vi "Write Field (Variant).vi"(7 "field name":string, 8 "error in (no error)":errorcluster, 10 "value in":variant, 11 "PV Data in":refnum<class "PV Data.lvclass">) -> (0 "error out":errorcluster, 2 "value out":variant, 3 "PV Data out":refnum<class "PV Data.lvclass">)   [LabVIEW 2020, in "PV Access.lvlib" / "PV Data.lvlib" / "PV Data.lvclass"]
uses:
  PV Data.lvclass
  <vilib>/ErrorRing/Error Ring.xnode
  PV Data.lvclass/PV Data.ctl
  cceb9e4b-eb75-48e8-aa55-ce9bdc72e988.vi
  c2285a35-9ffd-4e7b-9c27-aea24fb1581d.vi
  9a7adfbc-dfd7-46c4-b075-4f0440b83174.vi
  1bea9b6c-c326-4b2e-8e3d-45bf733a9c38.vi
  d9fbc47b-4e38-408d-93dd-f03e8c927dfc.vi
  878da8d4-af84-4ac8-b8bd-4e3d6f536ca0.vi
  22b99ade-ebf6-47b9-88b0-a2a84584e77c.vi
  7938dc55-06bb-4f46-98b4-31ec94e48f5a.vi
  17bcbbb4-445b-4ae2-9ca0-bb438421ceb4.vi
  76e53dd5-f0c3-4a89-968d-82371d9cf6ec.vi
  9c6bba7f-697c-4d5e-a550-b75ffba85a50.vi
  02c85caf-8b62-432b-a175-5fdc5c038fcc.vi
  5a5bdb7c-77ef-45fb-97e8-dbe02cadd076.vi
  b370053f-91cb-4be5-8525-cb241afcd6fe.vi
  a549df2c-920d-4323-ba7c-d4da420400e8.vi
  79192ce2-8dd6-4a70-8822-a4eb65a6aaee.vi
  1431eaa6-23a1-45b9-a4a3-2693041a1402.vi
  05adf883-15cd-45cb-9d7e-7746134da8fa.vi
  2414d7e0-05f5-4190-ab07-d4c7ba67c6a6.vi
  efa8a1d7-3bed-4705-901c-3918d28cffa5.vi
  26f11cd7-ec94-4004-9a33-110acaed2e3e.vi
  cc62e3b5-8986-4e79-a38c-535dac47f5c9.vi
  21c48d27-f92c-4ff3-9f7e-da22303d9520.vi
  0dfc8336-85bc-4349-aa6f-77eea7d3ae68.vi
  PV Data.lvlib
  <vilib>/Utility/Data Type/NI_Data Type.lvlib
  <vilib>/Utility/error.llb/Error Cluster From Error Code.vi
  Write Field (Boolean).vi
  Write Field (Boolean Array).vi
  Write Field (I8).vi
  Write Field (I8 Array).vi
  Write Field (I16).vi
  Write Field (I16 Array).vi
  Write Field (I32).vi
  Write Field (I32 Array).vi
  Write Field (I64).vi
  Write Field (I64 Array).vi
  Write Field (U8).vi
  Write Field (U8 Array).vi
  Write Field (U16).vi
  Write Field (U16 Array).vi
  Write Field (U32).vi
  Write Field (U32 Array).vi
  Write Field (U64).vi
  Write Field (U64 Array).vi
  Write Field (SGL).vi
  Write Field (DBL).vi
  Write Field (SGL Array).vi
  Write Field (DBL Array).vi
  Write Field (String).vi
  Write Field (String Array).vi
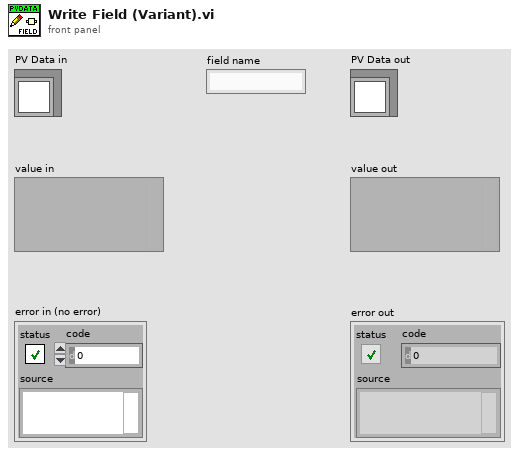
[diagram p1: front panel]
types:
  T1 = typedef "NI_Data Type.lvlib/Data Type.ctl" = enum8{"Invalid Type", "Void", "I8", "I16", "I32", "I64", "U8", "U16", "U32", "U64", "Single Float", "Double Float", "Extended Float", "Single Complex", "Double Complex", "Extended Complex", "Enum U8", "Enum U16", "Enum U32", "Enum U64", "Single Float With Unit", "Double Float With Unit", "Extended Float With Unit", "Single Complex with Unit", "Double Complex with Unit", "Extended Complex with Unit", "Boolean", "String", "Path", "Picture", "Tag", "Array", "Cluster", "Variant", "LV Variant", "Waveform", "Timestamp", "Digital Waveform", "Digital Data", "ExpressData", "Refnum", "External Data", "VI", "Poly VI", "LabVIEW Class Instance", "Fixed Point", "Set Collection", "Map Collection"}
  T2 = typedef "PV Access.lvlib/PV Data.lvlib/Type Code.ctl" = enum8{"Null", "Bool", "BoolA", "Int8", "Int8A", "Int16", "Int16A", "Int32", "Int32A", "Int64", "Int64A", "UInt8", "UInt8A", "UInt16", "UInt16A", "UInt32", "UInt32A", "UInt64", "UInt64A", "Float32", "Float32A", "Float64", "Float64A", "String", "StringA", "Struct", "StructA", "Union", "UnionA", "Any", "AnyA"}
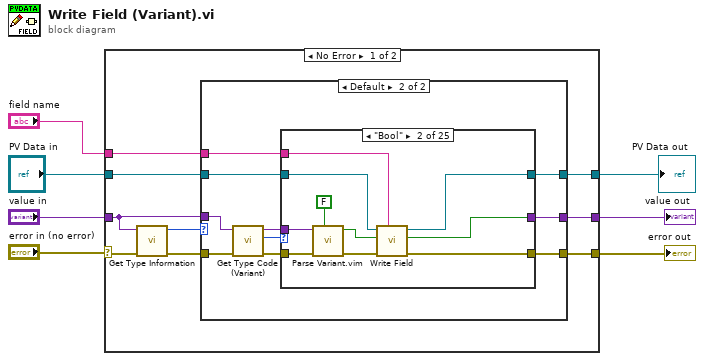
[diagram p0: block diagram]
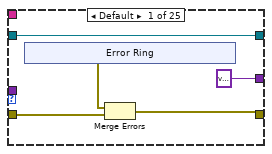
[diagram p3: hidden frame]
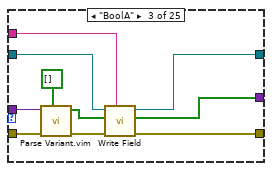
[diagram p4: hidden frame]
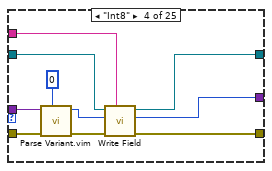
[diagram p5: hidden frame]
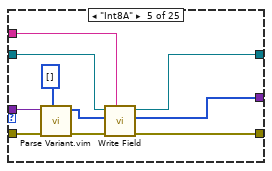
[diagram p6: hidden frame]
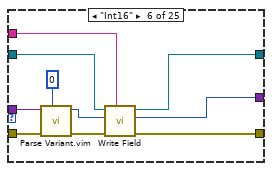
[diagram p7: hidden frame]
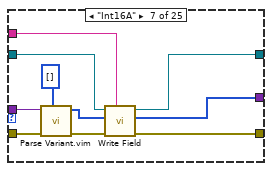
[diagram p8: hidden frame]
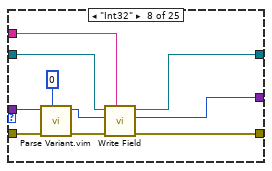
[diagram p9: hidden frame]
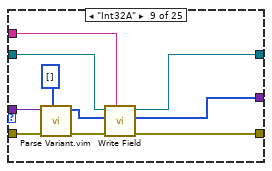
[diagram p10: hidden frame]
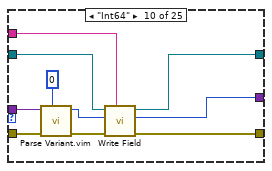
[diagram p11: hidden frame]
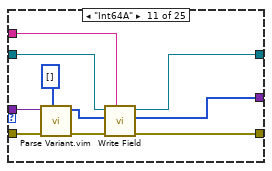
[diagram p12: hidden frame]
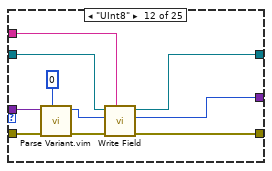
[diagram p13: hidden frame]
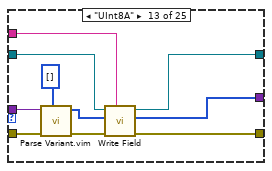
[diagram p14: hidden frame]
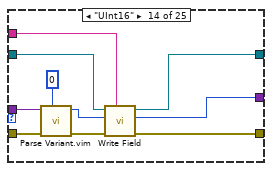
[diagram p15: hidden frame]
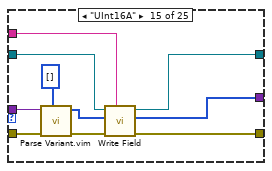
[diagram p16: hidden frame]
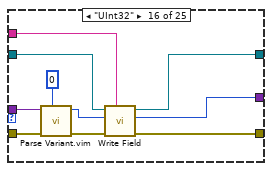
[diagram p17: hidden frame]
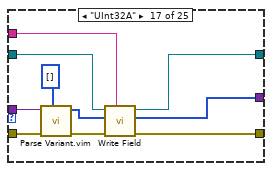
[diagram p18: hidden frame]
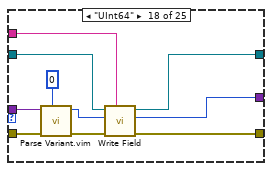
[diagram p19: hidden frame]
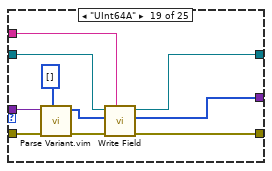
[diagram p20: hidden frame]
diagram:
  n1 = case shown="No Error" "error in (no error)" {
    selector: "error in (no error)" -> [w10 w279]
    tunnel: "value in" -> [w11 w280]
    tunnel: [w16 w280] -> w5
    tunnel: [w15 w279] -> w4
    tunnel: "PV Data in" -> [w14 w281]
    tunnel: [w13 w281] -> w2
    tunnel: "field name" -> [w12 _]
    frame No Error {
      n2 = call <vilib>:"Get Type Information.vi"("error in (no error)"=w10, "variant"=w11) -> ("error out"=w9:errorcluster, "type"=w8:T1)  [unwired: 5 in, 3 out]
      n3 = case shown="Default" w8 {
        tunnel: [w19 w26] -> w16
        tunnel: [w18 w25] -> w15
        tunnel: w14 -> [w17 w24]
        tunnel: [w17 w23] -> w13
        tunnel: w12 -> [_ w22]
        tunnel: w11 -> [w19 w21]
        tunnel: w9 -> [w18 w20]
        frame "Void" {
          # "Ignore void variants"
        }
        frame Default {
          n4 = call "Get Type Code (Variant).vi"("error in (no error)"=w20, "value"=w21) -> ("error out"=w27:errorcluster, "type code"=w29:T2, "value dup"=w28:variant)  [unwired: 5 in]
          n5 = case shown="\"Bool\"" w29 {
            tunnel: [w33 w45 w56 w66 w76 w86 w96 w106 w116 w126 w137 w146 w156 w166 w176 w186 w196 w206 w216 w226 w236 w246 w256 w266 w276] -> w25
            tunnel: w27 -> [w34 w48 w58 w68 w78 w88 w98 w108 w118 w128 w138 w148 w158 w168 w178 w188 w198 w208 w218 w228 w238 w248 w258 w268 w278]
            tunnel: [w30 w43 w54 w65 w74 w84 w94 w104 w114 w124 w135 w144 w154 w165 w174 w184 w195 w204 w214 w224 w234 w244 w254 w264 w274] -> w23
            tunnel: w28 -> [_ w42 w53 w64 w73 w83 w93 w103 w113 w123 w134 w143 w153 w164 w173 w183 w194 w203 w213 w223 w233 w243 w253 w263 w273]
            tunnel: [variant w41 w51 w62 w71 w81 w91 w101 w111 w121 w132 w141 w151 w162 w171 w181 w192 w201 w211 w221 w231 w241 w251 w261 w271] -> w26
            tunnel: w24 -> [w30 w40 w50 w61 w70 w80 w90 w100 w110 w120 w130 w140 w150 w161 w170 w180 w191 w200 w210 w220 w230 w240 w250 w259 w270]
            tunnel: w22 -> [_ w39 w49 w59 w69 w79 w89 w99 w109 w119 w129 w139 w149 w159 w169 w179 w189 w199 w209 w219 w229 w239 w249 w260 w269]
            frame Default {
              n6 = xnode "Error Ring"() -> ("error out"=w32:errorcluster)
              n7 = Merge Errors(w32, w34) -> (w33:errorcluster)
            }
            frame "Bool" {
              n8 = call "Parse Variant.vim"("default"=FALSE, "error in (no error)"=w48, "value"=w42) -> ("error out"=w46:errorcluster, "value out"=w44:bool)  [unwired: 7 in]
              n9 = call-poly "Write Field.vi"("field name"=w39, "error in"=w46, "value"=w44, "PV Data in"=w40) -> ("error out"=w45:errorcluster, "value out"=w41:bool, "PV Data out"=w43:refnum<class "PV Data.lvclass">)  [unwired: 5 in]
            }
            frame "BoolA" {
              n10 = call "Parse Variant.vim"("default"=bool[] [], "error in (no error)"=w58, "value"=w53) -> ("error out"=w57:errorcluster, "value out"=w55:bool[])  [unwired: 7 in]
              n11 = call-poly "Write Field.vi"("field name"=w49, "error in"=w57, "value"=w55, "PV Data in"=w50) -> ("error out"=w56:errorcluster, "value out"=w51:bool[], "PV Data out"=w54:refnum<class "PV Data.lvclass">)  [unwired: 5 in]
            }
            frame "Int8" {
              n12 = call "Parse Variant.vim"("default"=i8 0, "error in (no error)"=w68, "value"=w64) -> ("error out"=w67:errorcluster, "value out"=w60:i8)  [unwired: 7 in]
              n13 = call-poly "Write Field.vi"("field name"=w59, "error in"=w67, "value"=w60, "PV Data in"=w61) -> ("error out"=w66:errorcluster, "value out"=w62:i8, "PV Data out"=w65:refnum<class "PV Data.lvclass">)  [unwired: 5 in]
            }
            frame "Int8A" {
              n14 = call "Parse Variant.vim"("default"=i8[] [], "error in (no error)"=w78, "value"=w73) -> ("error out"=w77:errorcluster, "value out"=w75:i8[])  [unwired: 7 in]
              n15 = call-poly "Write Field.vi"("field name"=w69, "error in"=w77, "value"=w75, "PV Data in"=w70) -> ("error out"=w76:errorcluster, "value out"=w71:i8[], "PV Data out"=w74:refnum<class "PV Data.lvclass">)  [unwired: 5 in]
            }
            frame "Int16" {
              n16 = call "Parse Variant.vim"("default"=i16 0, "error in (no error)"=w88, "value"=w83) -> ("error out"=w87:errorcluster, "value out"=w85:i16)  [unwired: 7 in]
              n17 = call-poly "Write Field.vi"("field name"=w79, "error in"=w87, "value"=w85, "PV Data in"=w80) -> ("error out"=w86:errorcluster, "value out"=w81:i16, "PV Data out"=w84:refnum<class "PV Data.lvclass">)  [unwired: 5 in]
            }
            frame "Int16A" {
              n18 = call "Parse Variant.vim"("default"=i16[] [], "error in (no error)"=w98, "value"=w93) -> ("error out"=w97:errorcluster, "value out"=w95:i16[])  [unwired: 7 in]
              n19 = call-poly "Write Field.vi"("field name"=w89, "error in"=w97, "value"=w95, "PV Data in"=w90) -> ("error out"=w96:errorcluster, "value out"=w91:i16[], "PV Data out"=w94:refnum<class "PV Data.lvclass">)  [unwired: 5 in]
            }
            frame "Int32" {
              n20 = call "Parse Variant.vim"("default"=0, "error in (no error)"=w108, "value"=w103) -> ("error out"=w107:errorcluster, "value out"=w105:i32)  [unwired: 7 in]
              n21 = call-poly "Write Field.vi"("field name"=w99, "error in"=w107, "value"=w105, "PV Data in"=w100) -> ("error out"=w106:errorcluster, "value out"=w101:i32, "PV Data out"=w104:refnum<class "PV Data.lvclass">)  [unwired: 5 in]
            }
            frame "Int32A" {
              n22 = call "Parse Variant.vim"("default"=i32[] [], "error in (no error)"=w118, "value"=w113) -> ("error out"=w117:errorcluster, "value out"=w115:i32[])  [unwired: 7 in]
              n23 = call-poly "Write Field.vi"("field name"=w109, "error in"=w117, "value"=w115, "PV Data in"=w110) -> ("error out"=w116:errorcluster, "value out"=w111:i32[], "PV Data out"=w114:refnum<class "PV Data.lvclass">)  [unwired: 5 in]
            }
            frame "Int64" {
              n24 = call "Parse Variant.vim"("default"=i64 0, "error in (no error)"=w128, "value"=w123) -> ("error out"=w127:errorcluster, "value out"=w125:i64)  [unwired: 7 in]
              n25 = call-poly "Write Field.vi"("field name"=w119, "error in"=w127, "value"=w125, "PV Data in"=w120) -> ("error out"=w126:errorcluster, "value out"=w121:i64, "PV Data out"=w124:refnum<class "PV Data.lvclass">)  [unwired: 5 in]
            }
            frame "Int64A" {
              n26 = call "Parse Variant.vim"("default"=i64[] [], "error in (no error)"=w138, "value"=w134) -> ("error out"=w131:errorcluster, "value out"=w136:i64[])  [unwired: 7 in]
              n27 = call-poly "Write Field.vi"("field name"=w129, "error in"=w131, "value"=w136, "PV Data in"=w130) -> ("error out"=w137:errorcluster, "value out"=w132:i64[], "PV Data out"=w135:refnum<class "PV Data.lvclass">)  [unwired: 5 in]
            }
            frame "UInt8" {
              n28 = call "Parse Variant.vim"("default"=u8 0, "error in (no error)"=w148, "value"=w143) -> ("error out"=w147:errorcluster, "value out"=w145:u8)  [unwired: 7 in]
              n29 = call-poly "Write Field.vi"("field name"=w139, "error in"=w147, "value"=w145, "PV Data in"=w140) -> ("error out"=w146:errorcluster, "value out"=w141:u8, "PV Data out"=w144:refnum<class "PV Data.lvclass">)  [unwired: 5 in]
            }
            frame "UInt8A" {
              n30 = call "Parse Variant.vim"("default"=u8[] [], "error in (no error)"=w158, "value"=w153) -> ("error out"=w157:errorcluster, "value out"=w155:u8[])  [unwired: 7 in]
              n31 = call-poly "Write Field.vi"("field name"=w149, "error in"=w157, "value"=w155, "PV Data in"=w150) -> ("error out"=w156:errorcluster, "value out"=w151:u8[], "PV Data out"=w154:refnum<class "PV Data.lvclass">)  [unwired: 5 in]
            }
            frame "UInt16" {
              n32 = call "Parse Variant.vim"("default"=u16 0, "error in (no error)"=w168, "value"=w164) -> ("error out"=w167:errorcluster, "value out"=w160:u16)  [unwired: 7 in]
              n33 = call-poly "Write Field.vi"("field name"=w159, "error in"=w167, "value"=w160, "PV Data in"=w161) -> ("error out"=w166:errorcluster, "value out"=w162:u16, "PV Data out"=w165:refnum<class "PV Data.lvclass">)  [unwired: 5 in]
            }
            frame "UInt16A" {
              n34 = call "Parse Variant.vim"("default"=u16[] [], "error in (no error)"=w178, "value"=w173) -> ("error out"=w177:errorcluster, "value out"=w175:u16[])  [unwired: 7 in]
              n35 = call-poly "Write Field.vi"("field name"=w169, "error in"=w177, "value"=w175, "PV Data in"=w170) -> ("error out"=w176:errorcluster, "value out"=w171:u16[], "PV Data out"=w174:refnum<class "PV Data.lvclass">)  [unwired: 5 in]
            }
            frame "UInt32" {
              n36 = call "Parse Variant.vim"("default"=u32 0, "error in (no error)"=w188, "value"=w183) -> ("error out"=w187:errorcluster, "value out"=w185:u32)  [unwired: 7 in]
              n37 = call-poly "Write Field.vi"("field name"=w179, "error in"=w187, "value"=w185, "PV Data in"=w180) -> ("error out"=w186:errorcluster, "value out"=w181:u32, "PV Data out"=w184:refnum<class "PV Data.lvclass">)  [unwired: 5 in]
            }
            frame "UInt32A" {
              n38 = call "Parse Variant.vim"("default"=u32[] [], "error in (no error)"=w198, "value"=w194) -> ("error out"=w197:errorcluster, "value out"=w190:u32[])  [unwired: 7 in]
              n39 = call-poly "Write Field.vi"("field name"=w189, "error in"=w197, "value"=w190, "PV Data in"=w191) -> ("error out"=w196:errorcluster, "value out"=w192:u32[], "PV Data out"=w195:refnum<class "PV Data.lvclass">)  [unwired: 5 in]
            }
            frame "UInt64" {
              n40 = call "Parse Variant.vim"("default"=u64 0, "error in (no error)"=w208, "value"=w203) -> ("error out"=w207:errorcluster, "value out"=w205:u64)  [unwired: 7 in]
              n41 = call-poly "Write Field.vi"("field name"=w199, "error in"=w207, "value"=w205, "PV Data in"=w200) -> ("error out"=w206:errorcluster, "value out"=w201:u64, "PV Data out"=w204:refnum<class "PV Data.lvclass">)  [unwired: 5 in]
            }
            frame "UInt64A" {
              n42 = call "Parse Variant.vim"("default"=u64[] [], "error in (no error)"=w218, "value"=w213) -> ("error out"=w217:errorcluster, "value out"=w215:u64[])  [unwired: 7 in]
              n43 = call-poly "Write Field.vi"("field name"=w209, "error in"=w217, "value"=w215, "PV Data in"=w210) -> ("error out"=w216:errorcluster, "value out"=w211:u64[], "PV Data out"=w214:refnum<class "PV Data.lvclass">)  [unwired: 5 in]
            }
            frame "Float32" {
              n44 = call "Parse Variant.vim"("default"=sgl 0.0, "error in (no error)"=w228, "value"=w223) -> ("error out"=w227:errorcluster, "value out"=w225:sgl)  [unwired: 7 in]
              n45 = call-poly "Write Field.vi"("field name"=w219, "error in"=w227, "value"=w225, "PV Data in"=w220) -> ("error out"=w226:errorcluster, "value out"=w221:sgl, "PV Data out"=w224:refnum<class "PV Data.lvclass">)  [unwired: 5 in]
            }
            frame "Float64" {
              n46 = call "Parse Variant.vim"("default"=0.0, "error in (no error)"=w238, "value"=w233) -> ("error out"=w237:errorcluster, "value out"=w235:dbl)  [unwired: 7 in]
              n47 = call-poly "Write Field.vi"("field name"=w229, "error in"=w237, "value"=w235, "PV Data in"=w230) -> ("error out"=w236:errorcluster, "value out"=w231:dbl, "PV Data out"=w234:refnum<class "PV Data.lvclass">)  [unwired: 5 in]
            }
            frame "Float32A" {
              n48 = call "Parse Variant.vim"("default"=sgl[] [], "error in (no error)"=w248, "value"=w243) -> ("error out"=w247:errorcluster, "value out"=w245:sgl[])  [unwired: 7 in]
              n49 = call-poly "Write Field.vi"("field name"=w239, "error in"=w247, "value"=w245, "PV Data in"=w240) -> ("error out"=w246:errorcluster, "value out"=w241:sgl[], "PV Data out"=w244:refnum<class "PV Data.lvclass">)  [unwired: 5 in]
            }
            frame "Float64A" {
              n50 = call "Parse Variant.vim"("default"=dbl[] [], "error in (no error)"=w258, "value"=w253) -> ("error out"=w257:errorcluster, "value out"=w255:dbl[])  [unwired: 7 in]
              n51 = call-poly "Write Field.vi"("field name"=w249, "error in"=w257, "value"=w255, "PV Data in"=w250) -> ("error out"=w256:errorcluster, "value out"=w251:dbl[], "PV Data out"=w254:refnum<class "PV Data.lvclass">)  [unwired: 5 in]
            }
            frame "String" {
              n52 = call "Parse Variant.vim"("default"="", "error in (no error)"=w268, "value"=w263) -> ("error out"=w267:errorcluster, "value out"=w265:string)  [unwired: 7 in]
              n53 = call-poly "Write Field.vi"("field name"=w260, "error in"=w267, "value"=w265, "PV Data in"=w259) -> ("error out"=w266:errorcluster, "value out"=w261:string, "PV Data out"=w264:refnum<class "PV Data.lvclass">)  [unwired: 5 in]
            }
            frame "StringA" {
              n54 = call "Parse Variant.vim"("default"=string[] [], "error in (no error)"=w278, "value"=w273) -> ("error out"=w277:errorcluster, "value out"=w275:string[])  [unwired: 7 in]
              n55 = call-poly "Write Field.vi"("field name"=w269, "error in"=w277, "value"=w275, "PV Data in"=w270) -> ("error out"=w276:errorcluster, "value out"=w271:string[], "PV Data out"=w274:refnum<class "PV Data.lvclass">)  [unwired: 5 in]
            }
          }
        }
      }
    }
    frame Error {
    }
  }
  "value out" <- w5
  "error out" <- w4
  "PV Data out" <- w2
